vi "Configure Device.vi"(8 "error in (no error)":errorcluster, 11 "Simulated Scope in":refnum<class "Simulated Scope.lvclass">) -> (0 "error out":errorcluster, 3 "Simulated Scope out":refnum<class "Simulated Scope.lvclass">)   [LabVIEW 2020, in "Simulated Scope.lvlib" / "Simulated Scope.lvclass"]
uses:
  Simulated Scope.lvclass
  Simulated Scope.lvclass/Simulated Scope.ctl
  build/ppl/lv-hal.lvlibp/Device/Device.lvclass
  C:/dev/HAL Demo/build/ppl/lv-hal.lvlibp/Device/Device.lvclass
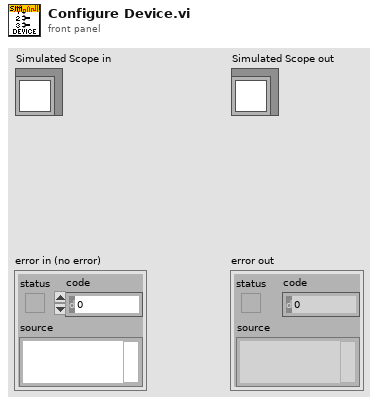
[diagram p1: front panel]
types:
  T1 = typedef "Simulated Scope.lvlib/Simulated Scope.lvclass/Ref Data.ctl" = cluster{"Sim Queue Name":string, "Waveform Queue":refnum<queue>}
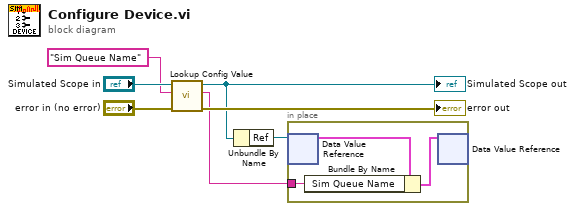
[diagram p0: block diagram]
diagram:
  n1 = call "Lookup Config Value.vi"("error in (no error)"="error in (no error)", "Config Key"="Sim Queue Name", "Device in"="Simulated Scope in") -> ("error out"=→"error out":errorcluster, "Value"=w1:string, "Device out"=w2:refnum<class "Simulated Scope.lvclass">)  [unwired: 5 in, 1 out]
  "Simulated Scope out" <- w2
  n2 = Unbundle By Name(w2) -> ("Ref"=w4:refnum<data-value>)
  n3 = in-place {
    in-place-border: w1 -> [w8]
    n4 = in-place-dvr #1(w4) -> (w10:T1)  [unwired: 1 out]
    n5 = Bundle By Name(cluster=w10, "Sim Queue Name"=w8) -> (w9:T1)
    n6 = in-place-dvr #1(w9) -> ()  [unwired: 2 out]
  }
